vi "01_Main.vi"() -> ()   [LabVIEW 2023]
doc: "This VI shows how to setup and execute a measurement without any user input."
panel:
  out "Loop Counter":i32
  out "size(s)":i32[](array[numeric])
  in  "Fahrprofil Datei":path
  out "IP-Adresse Antrieb":string="192.168.10.5"
  in  "BETRIEBSART ANTRIEB":bool
  in  "Motoren":bool
  out "Digital Antrieb":dbl
  out "Drehmoment Antrieb":dbl
  out "Status/Fehler Antrieb":dbl
  out "Istgeschwindigkeit Antrieb":dbl
  in  "Digital Antrieb":dbl
  in  "Deceleration Antrieb":dbl
  in  "Acceleration Antrieb":dbl
  in  "Speed Antrieb":dbl
  out "IP-Adresse Last":string
  out "Digital":dbl
  out "Drehmoment":dbl
  out "Status/Fehler":dbl
  out "Istgeschwindigkeit":dbl
  in  "Digital A":dbl
  in  "Deceleration":dbl
  in  "Acceleration":dbl
  in  "Speed":dbl
  out "Reserviert":bool
  out "SWES inaktiv":bool
  out "Geschwindigkeit erreicht":bool
  out "Warnung":bool
  out "Fehler":bool
  out "in Position":bool
  out "Relativposition übernommen":bool
  out "Motor dreht":bool
  out "Bremse geöffnet":bool
  out "Endstufenfreigabe":bool
  out "STO inaktiv":bool
  out "Betriebsbereit":bool
  out "Reserviert 8":bool
  out "SWES inaktiv 2":bool
  out "Geschwindigkeit erreicht 2":bool
  out "Warnung 2":bool
  out "Fehler 2":bool
  out "in Position 2":bool
  out "Relativposition übernommen 2":bool
  out "Motor dreht 2":bool
  out "Bremse geöffnet 2":bool
  out "Endstufenfreigabe 2":bool
  out "STO inaktiv 2":bool
  out "Betriebsbereit 2":bool
  in  "Reserviert 9":bool
  in  "Reservier 2":bool
  in  "Reserviert 10":bool
  in  "Reserviert 11":bool
  in  "Reserviert 12":bool
  in  "Reserviert 13":bool
  in  "Reserviert 14":bool
  in  "Reserviert 2":bool
  in  "Reservier":bool
  in  "Reserviert 3":bool
  in  "Reserviert 4":bool
  in  "Reserviert 5":bool
  in  "Reserviert 6":bool
  in  "Reserviert 7":bool
  in  "Bedienelemente - Lastmotor":enum32{"Standard", "Versteckt"}(tab)
  in  "Enable/EmergencyStop Antrieb":bool
  in  "Fehler_Reset Antrieb":bool
  in  "Start L":bool
  in  "Enable/ApplicationStop Antrieb":bool
  in  "Inhibit L":bool
  in  "Standby Antrieb":bool
  in  "Handshake Antrieb":bool
  in  "AS2 aktivieren Antrieb":bool
  in  "Bremse öffnen Antrieb":bool
  out "Standby aktiv 2":bool
  out "AS2 aktiv 2":bool
  out "Handshake 3":bool
  out "referenziert 2":bool
  in  "Bedienelemente - Antriebsmotor":enum32{"Standard", "Versteckt"}(tab)
  in  "Enable/EmergencyStop":bool
  in  "Enable/ApplicationStop":bool
  in  "Fehler_Reset":bool
  in  "Start":bool
  in  "Inhibit":bool
  in  "Standby":bool
  in  "Handshake 2":bool
  in  "AS2 aktivieren":bool
  in  "Bremse öffnen":bool
  out "AS2 aktiv":bool
  out "Handshake":bool
  out "Standby aktiv":bool
  out "referenziert":bool
  out "Numeric":i32
  out "VI wird beendet":string
  in  "VI-Stopp":bool
  out "Diagram 2":waveform(dbl)(graph)
  in  "Kanal 2":i32=2 min=1 max=4 step=1
  in  "Kanal":i32=1 min=1 max=4 step=1
  in  "Datei-Pfad":path
  out "Diagram":waveform(dbl)(graph)
  in  "Messung":bool=TRUE
  out "HBM Driver\nLicense is valid":bool
  # "Betriebsart des Antrieb-Motors wählen; Wenn ein Fahrprofil geladen werden soll dieses über die Datei-Auswahl auswählen. \n\nDanach die Ansteuerung der Motoren mit BETRIEBSART BESTÄTIGEN starten."
  # "Handbetrieb"
  # "Fahrprofil laden"
  # "Manuelle Ansteuerung des Last-Motors"
  # "Manuelle Ansteuerung des Antrieb-Motors"
  # "Datenaquise mit dem HBM Messverstärker"
  # "Messung mit START starten.\n\nWenn die Messdaten gespeichert werden sollen, muss vor \ndem Starten der Messung ein gültiger Dateipfad angegeben werden."
  # "Datenaufzeichnung"
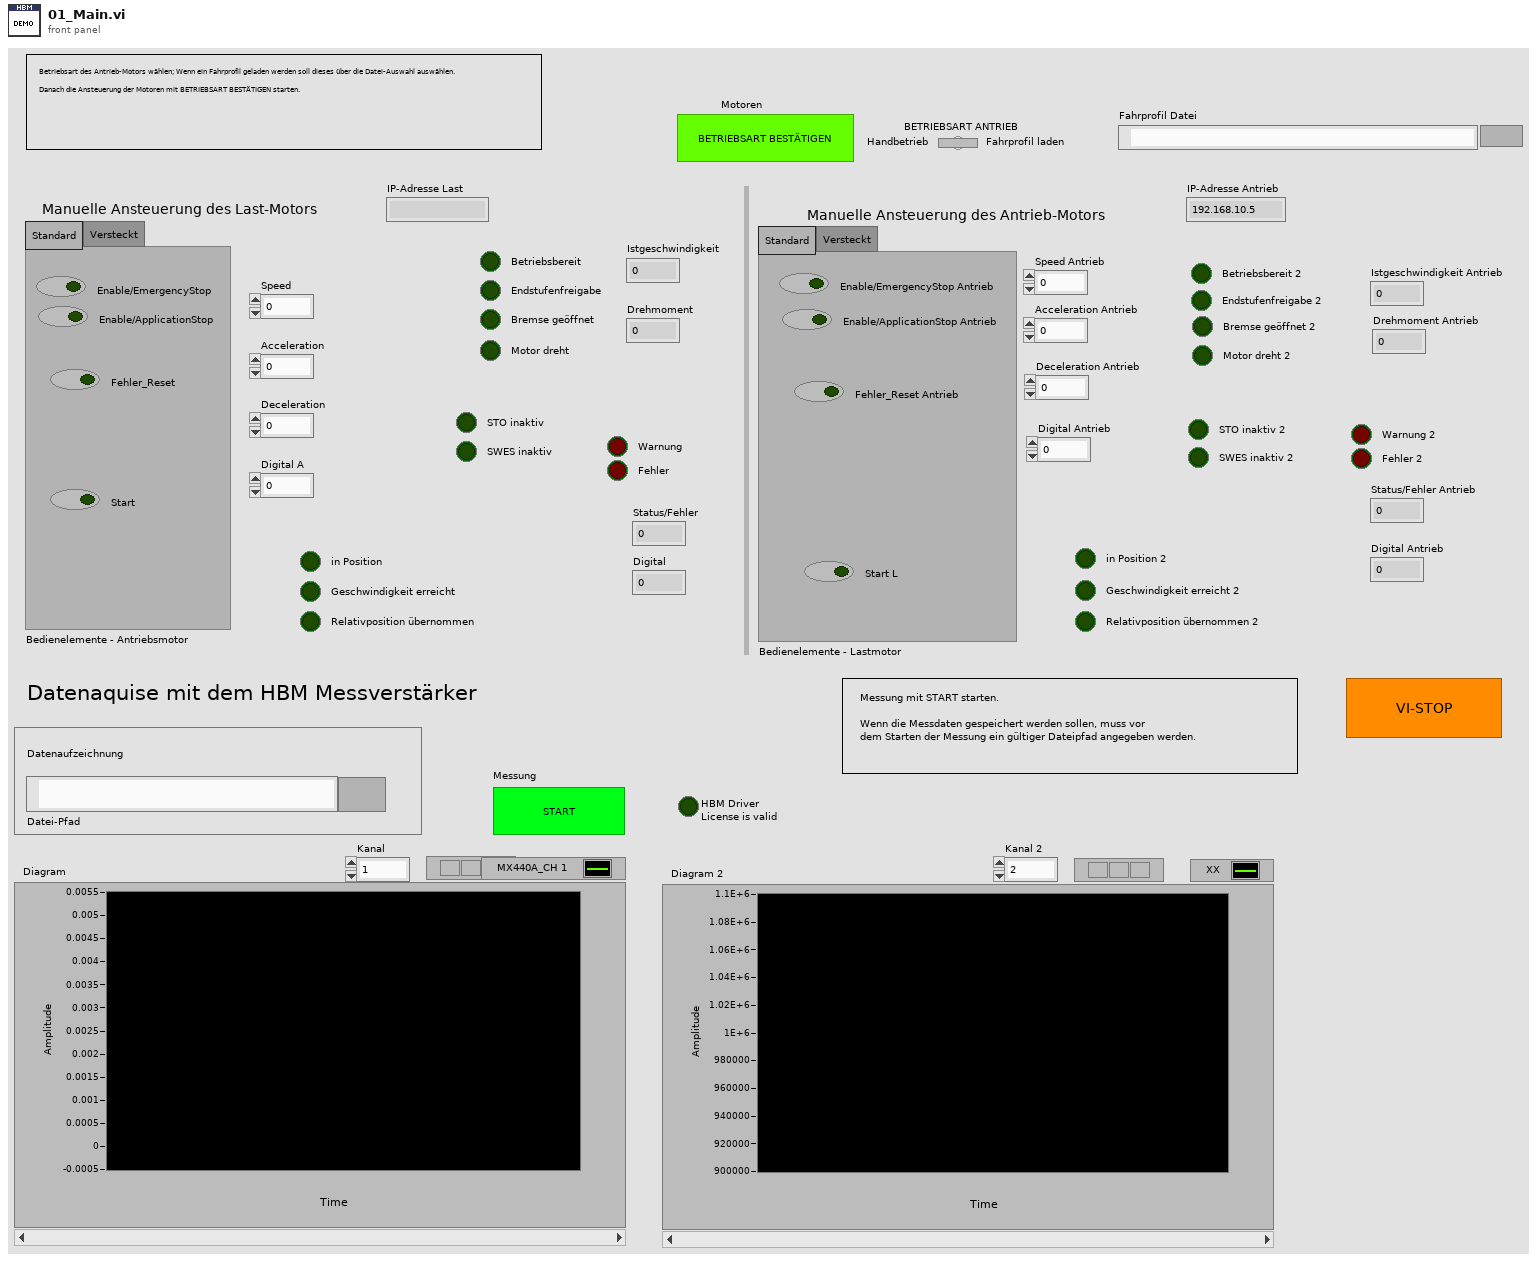
[diagram p1: front panel]
types:
  T1 = cluster{"Devices":refnum<k24>[], "Signals":refnum<k24>[]}
  T2 = enum16{"open", "replace", "create", "open or create", "replace or create", "replace or create with confirmation"}
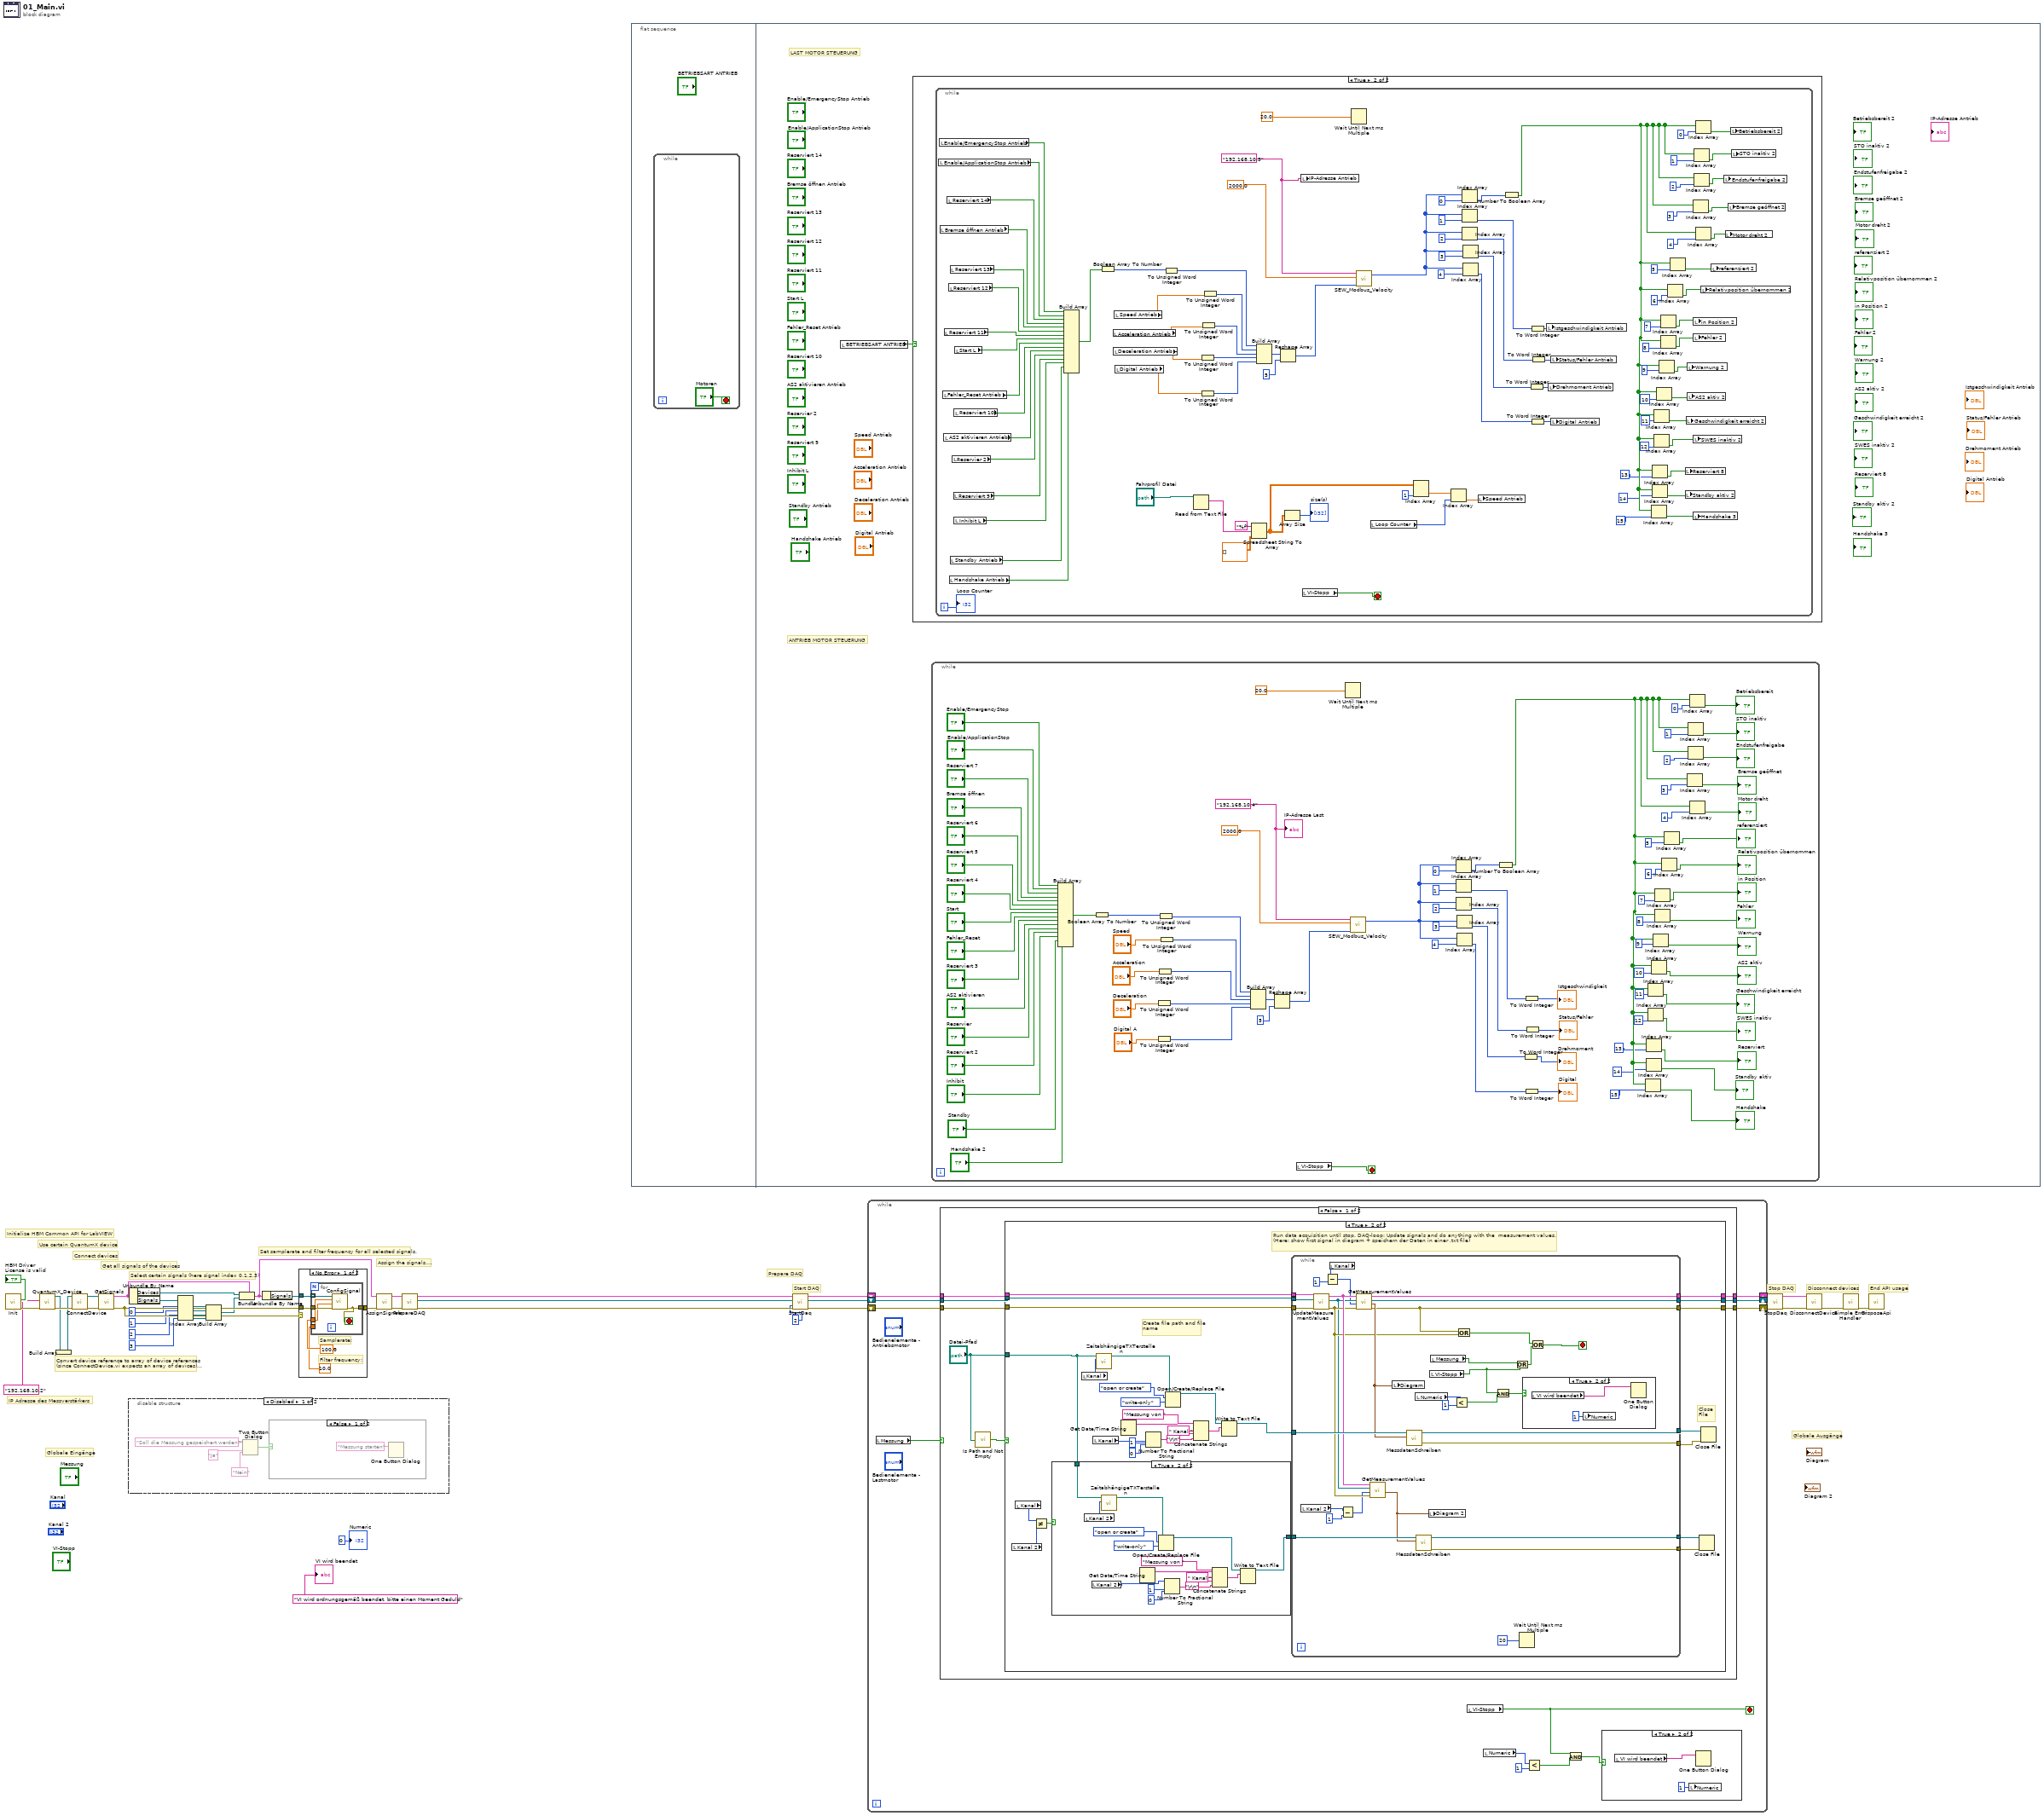
[diagram p0: block diagram]
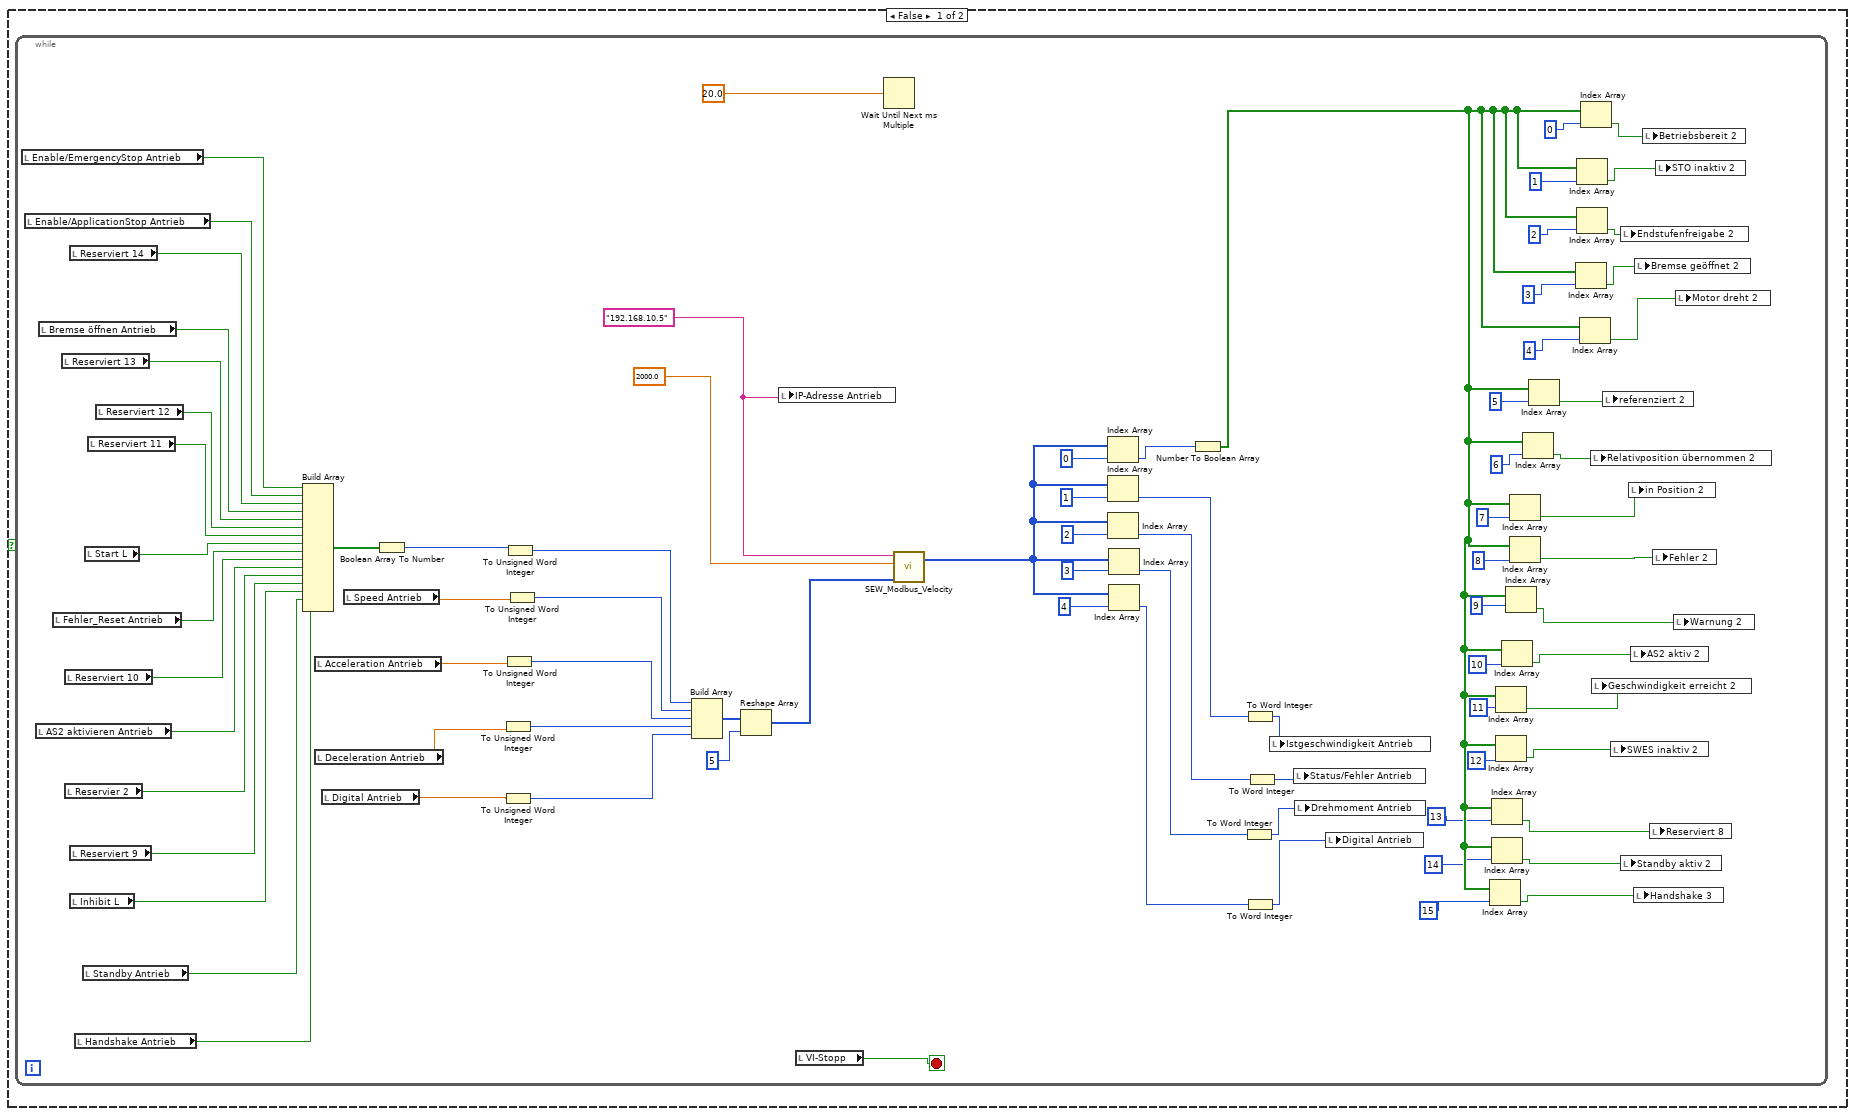
[diagram p2: hidden frame]
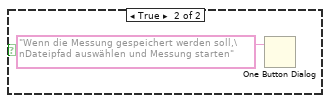
[diagram p3: hidden frame]
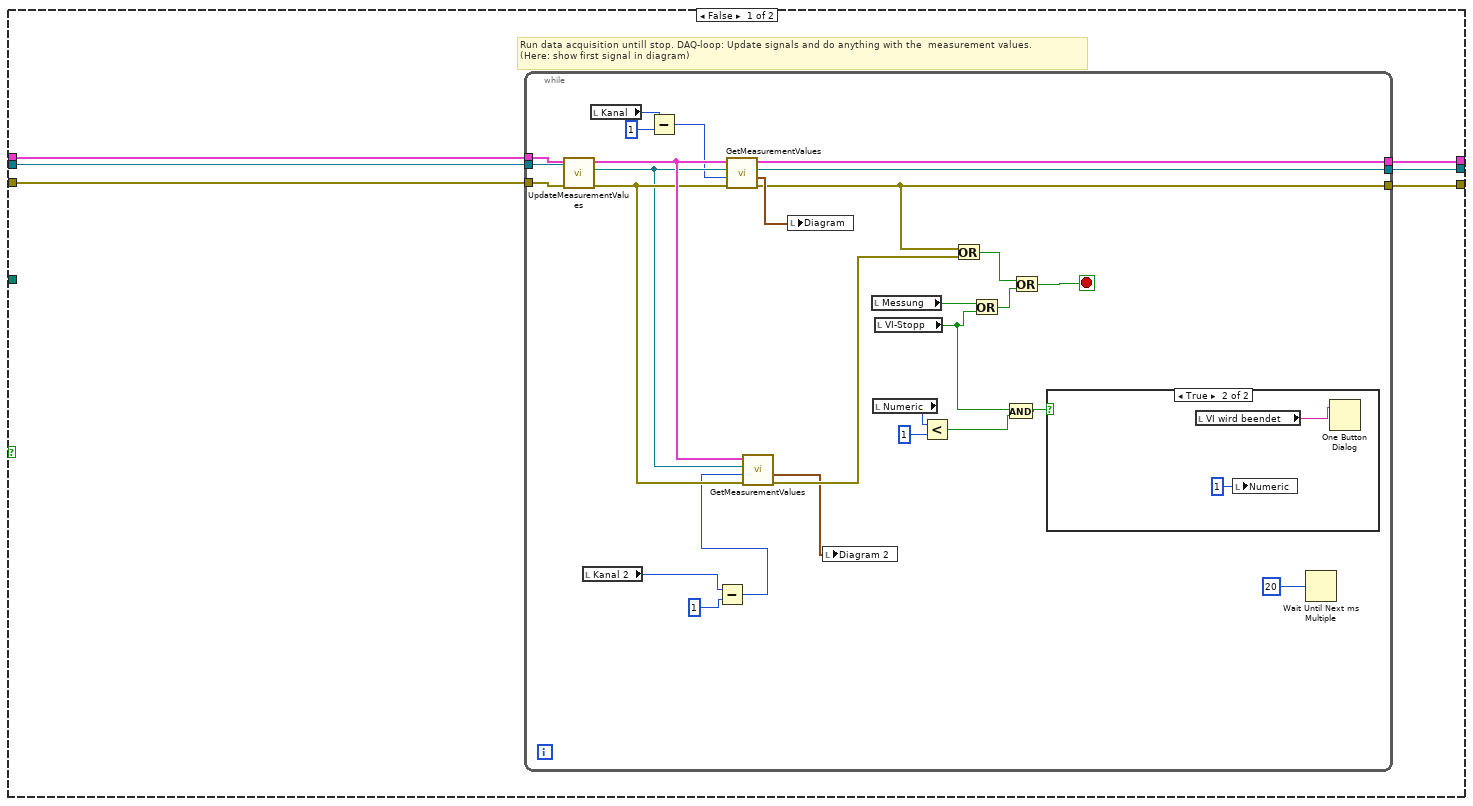
[diagram p6: hidden frame]
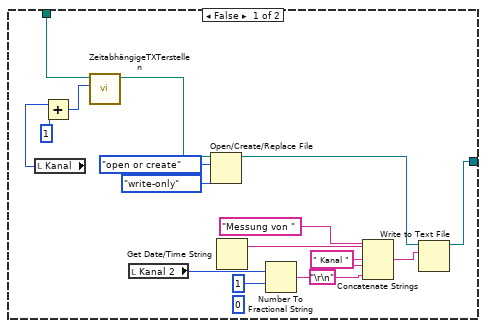
[diagram p8: hidden frame]
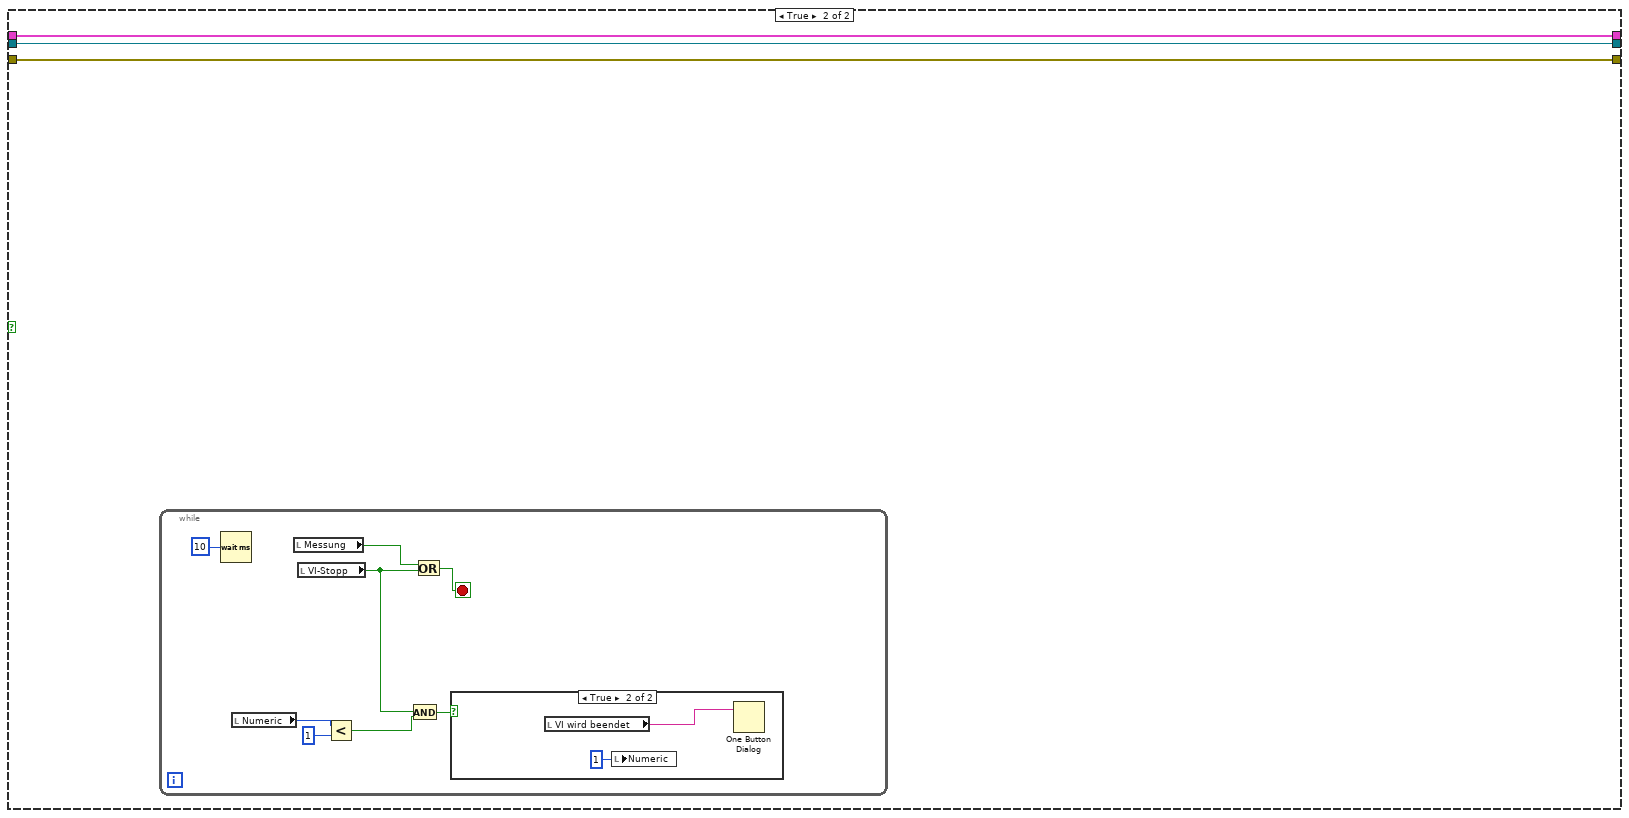
[diagram p10: hidden frame]
diagram:
  # "Globale Ausgänge"
  # "Globale Eingänge"
  # "IP Adresse des Messverstärkers"
  # "Convert device reference to array of device references\n(since ConnectDevice.vi expects an array of devices)..."
  # "Disconnect devices"
  # "Set samplerate and filter frequency for all selected signals."
  # "Initialize HBM Common API for LabVIEW"
  # "End API usage"
  # "Stop DAQ"
  # "Start DAQ"
  # "Prepare DAQ"
  # "Select certain signals (here signal index 0,1,2,3)"
  # "Get all signals of the devices"
  # "Connect devices"
  # "Use certain QuantumX device"
  # "Assign the signals...."
  n1 = call "Init.vi"() -> ("LicenseIsValid"=→"HBM Driver\nLicense is valid":bool, "Error out"=w12:errorcluster)  [unwired: 8 in, 1 out]
  n2 = call "QuantumX_Device.vi"("Error in"=w12, "IPAddress"="192.168.10.2" ("IPAddress of QuantumX device")) -> ("Error out"=w13:errorcluster, "Device"=w10:refnum<k24>)  [unwired: 6 in]
  n3 = Build Array(w10) -> (w9:refnum<k24>[])
  n4 = call "ConnectDevice.vi"("Error in"=w13, "Devices"=w9) -> ("Error out"=w35:errorcluster, "Devices"=w34:refnum<k24>[])  [unwired: 7 in, 1 out]
  n5 = call "GetSignals.vi"("Error in"=w35, "Devices"=w34) -> ("Error out"=w29:errorcluster, "DevicesAndSignals"=w30:T1)  [unwired: 8 in]
  n6 = disable-structure shown="Disabled" {
    frame Disabled {
      n7 = Two Button Dialog(message="Soll die Messung gespeichert werden?", 1:"Nein" ("F button name (\"Cancel\")"), 2:"Ja" ("T button name (\"OK\")")) -> (T button?=w46:bool)
      n8 = case shown="False" w46 {
        frame False {
          n9 = One Button Dialog(message="Messung starten") -> ()  [unwired: 1 in, 1 out]
        }
        frame True {
          n10 = One Button Dialog(message="Wenn die Messung gespeichert werden soll,\nDateipfad auswählen und Messung starten") -> ()  [unwired: 1 in, 1 out]
        }
      }
    }
    frame Enabled {
    }
  }
  n11 = Unbundle By Name(w30) -> ("Devices"=w23:refnum<k24>[], "Signals"=w27:refnum<k24>[])
  n12 = Index Array(array=w27, index #1=0 ("Index"), index #2=1 ("Index"), index #3=2 ("Index"), index #4=3 ("Index")) -> (element #1=w26:refnum<k24>, element #2=w25:refnum<k24>, element #3=w18:refnum<k24>, element #4=w17:refnum<k24>)
  n13 = Build Array(w26, w25, w18, w17) -> (w24:refnum<k24>[])
  n14 = Bundle(cluster=w30, "Devices"=w23, "Signals"=w24) -> (w31:T1)
  n15 = Unbundle By Name(w31) -> ("Signals"=w42:refnum<k24>[])
  n16 = case shown="No Error" w29 {
    tunnel: w29 -> [w53 w59]
    tunnel: w42 -> [w52 _]
    tunnel: [w51 w59] -> w41
    frame No Error {
      # "Filter frequency:"
      # "Samplerate:"
      n17 = for {
        tunnel: w53 -> [w58]
        tunnel: 100.0 ("SampleRate") -> [w57]
        tunnel: 10.0 ("FilterFrequency") -> [w56]
        tunnel: w52 -> [w55] mode=indexing
        tunnel: [w54] -> w51
        stop <- w54 stop-if-true
        n18 = call "ConfigSignal.vi"("Error in"=w58, "SampleRate"=w57, "FilterFrequency"=w56, "Signal"=w55) -> ("Error out"=w54:errorcluster)  [unwired: 7 in]
      }
    }
    frame Error {
    }
  }
  n19 = call "AssignSignals.vi"("Error in"=w41, "DevicesAndSignals"=w31) -> ("Error out"=w39:errorcluster, "DevicesAndSignals"=w40:T1)  [unwired: 8 in]
  n20 = call "PrepareDAQ.vi"("Error in"=w39, "DevicesAndSignals"=w40) -> ("Error out"=w36:errorcluster, "DaqMeasurement"=w37:refnum<k24>, "DevicesAndSignals"=w38:T1)  [unwired: 7 in]
  n21 = flat-sequence {
    frame #0 {
      n22 = while {
        stop <- "Motoren" stop-if-true
      }
    }
    frame #1 {
      # "ANTRIEB MOTOR STEUERUNG"
      # "LAST MOTOR STEUERUNG"
      n23 = local read "BETRIEBSART ANTRIEB"() -> (w61:bool)
      n24 = case shown="True" w61 {
        frame False {
          n25 = while {
            stop <- w103 stop-if-true
            w62 = "192.168.10.5"
            n26 = local read "Enable/EmergencyStop Antrieb"() -> (w86:bool)
            n27 = local read "Enable/ApplicationStop Antrieb"() -> (w85:bool)
            n28 = local read "AS2 aktivieren Antrieb"() -> (w75:bool)
            n29 = local read "Bremse öffnen Antrieb"() -> (w83:bool)
            n30 = local read "Fehler_Reset Antrieb"() -> (w74:bool)
            n31 = local read "Reserviert 13"() -> (w82:bool)
            n32 = local read "Reserviert 10"() -> (w77:bool)
            n33 = local read "Reservier 2"() -> (w76:bool)
            n34 = local read "Reserviert 14"() -> (w84:bool)
            n35 = local read "Reserviert 9"() -> (w78:bool)
            n36 = local read "Inhibit L"() -> (w79:bool)
            n37 = local read "Handshake Antrieb"() -> (w81:bool)
            n38 = local read "Standby Antrieb"() -> (w80:bool)
            n39 = local read "Start L"() -> (w73:bool)
            n40 = local read "Reserviert 11"() -> (w72:bool)
            n41 = local read "Reserviert 12"() -> (w71:bool)
            n42 = Build Array(w86, w85, w84, w83, w82, w71, w72, w73, w74, w77, w75, w76, w78, w79, w80, w81) -> (w136:bool[])
            n43 = local read "Acceleration Antrieb"() -> (w65:dbl)
            n44 = local read "Deceleration Antrieb"() -> (w64:dbl)
            n45 = local read "Digital Antrieb"() -> (w63:dbl)
            n46 = local read "Speed Antrieb"() -> (w66:dbl)
            n47 = Boolean Array To Number(Boolean array=w136) -> (number=w137:u32)
            n48 = To Unsigned Word Integer(number=w64) -> (unsigned 16bit integer=w140:u16)
            n49 = To Unsigned Word Integer(number=w63) -> (unsigned 16bit integer=w141:u16)
            n50 = To Unsigned Word Integer(number=w65) -> (unsigned 16bit integer=w139:u16)
            n51 = To Unsigned Word Integer(number=w137) -> (unsigned 16bit integer=w138:u16)
            n52 = To Unsigned Word Integer(number=w66) -> (unsigned 16bit integer=w142:u16)
            n53 = Build Array(w138, w142, w139, w140, w141) -> (w143:u16[])
            n54 = Reshape Array(w143, 5) -> (w133:u16[])
            n55 = local write "IP-Adresse Antrieb"(w62) -> ()
            n56 = local read "VI-Stopp"() -> (w103:bool)
            n57 = Wait Until Next ms Multiple(millisecond multiple=20.0 ("Update(ms)")) -> ()  [unwired: 1 out]
            n58 = call "SEW_Modbus_Velocity.vi"("Remote IP Address"=w62, "Timeout [ms]"=2000.0 ("Timeout (ms)"), "Output (Write Multiple Register) 2"=w133) -> ("Input (Read Holding Register) 2"=w131:u16[])  [unwired: 3 in]
            n59 = Index Array(array=w131, index=0) -> (element=w121:u16)
            n60 = Index Array(array=w131, index=1) -> (element=w122:u16)
            n61 = Index Array(array=w131, index=2) -> (element=w123:u16)
            n62 = Index Array(array=w131, index=3) -> (element=w124:u16)
            n63 = Index Array(array=w131, index=4) -> (element=w125:u16)
            n64 = Number To Boolean Array(number=w121) -> (Boolean array=w120:bool[])
            n65 = To Word Integer(number=w124) -> (16bit integer=w68:i16)
            n66 = To Word Integer(number=w122) -> (16bit integer=w70:i16)
            n67 = To Word Integer(number=w125) -> (16bit integer=w67:i16)
            n68 = To Word Integer(number=w123) -> (16bit integer=w69:i16)
            n69 = local write "Istgeschwindigkeit Antrieb"(w70) -> ()
            n70 = local write "Status/Fehler Antrieb"(w69) -> ()
            n71 = local write "Drehmoment Antrieb"(w68) -> ()
            n72 = local write "Digital Antrieb"(w67) -> ()
            n73 = Index Array(array=w120, index=15) -> (element=w87:bool)
            n74 = Index Array(array=w120, index=13) -> (element=w89:bool)
            n75 = Index Array(array=w120, index=14) -> (element=w88:bool)
            n76 = Index Array(array=w120, index=11) -> (element=w91:bool)
            n77 = Index Array(array=w120, index=12) -> (element=w90:bool)
            n78 = Index Array(array=w120, index=10) -> (element=w92:bool)
            n79 = Index Array(array=w120, index=9) -> (element=w93:bool)
            n80 = Index Array(array=w120, index=7) -> (element=w95:bool)
            n81 = Index Array(array=w120, index=8) -> (element=w94:bool)
            n82 = Index Array(array=w120, index=6) -> (element=w96:bool)
            n83 = Index Array(array=w120, index=5) -> (element=w97:bool)
            n84 = Index Array(array=w120, index=3) -> (element=w99:bool)
            n85 = Index Array(array=w120, index=1) -> (element=w101:bool)
            n86 = Index Array(array=w120, index=2) -> (element=w100:bool)
            n87 = Index Array(array=w120, index=4) -> (element=w98:bool)
            n88 = Index Array(array=w120, index=0) -> (element=w102:bool)
            n89 = local write "Relativposition übernommen 2"(w96) -> ()
            n90 = local write "Geschwindigkeit erreicht 2"(w91) -> ()
            n91 = local write "referenziert 2"(w97) -> ()
            n92 = local write "SWES inaktiv 2"(w90) -> ()
            n93 = local write "Endstufenfreigabe 2"(w100) -> ()
            n94 = local write "Standby aktiv 2"(w88) -> ()
            n95 = local write "in Position 2"(w95) -> ()
            n96 = local write "AS2 aktiv 2"(w92) -> ()
            n97 = local write "Handshake 3"(w87) -> ()
            n98 = local write "Bremse geöffnet 2"(w99) -> ()
            n99 = local write "Betriebsbereit 2"(w102) -> ()
            n100 = local write "Reserviert 8"(w89) -> ()
            n101 = local write "Fehler 2"(w94) -> ()
            n102 = local write "STO inaktiv 2"(w101) -> ()
            n103 = local write "Warnung 2"(w93) -> ()
            n104 = local write "Motor dreht 2"(w98) -> ()
          }
        }
        frame True {
          n105 = while {
            i -> [w146]
            stop <- w196 stop-if-true
            w155 = "192.168.10.5"
            n106 = local read "Enable/ApplicationStop Antrieb"() -> (w177:bool)
            n107 = local read "Enable/EmergencyStop Antrieb"() -> (w176:bool)
            n108 = local read "Bremse öffnen Antrieb"() -> (w179:bool)
            n109 = local read "Fehler_Reset Antrieb"() -> (w184:bool)
            n110 = local read "AS2 aktivieren Antrieb"() -> (w186:bool)
            n111 = local read "Reserviert 11"() -> (w182:bool)
            n112 = local read "Reserviert 14"() -> (w178:bool)
            n113 = local read "Reserviert 12"() -> (w181:bool)
            n114 = local read "Handshake Antrieb"() -> (w191:bool)
            n115 = local read "Reserviert 13"() -> (w180:bool)
            n116 = local read "Standby Antrieb"() -> (w190:bool)
            n117 = local read "Reservier 2"() -> (w187:bool)
            n118 = local read "Reserviert 9"() -> (w188:bool)
            n119 = local read "Reserviert 10"() -> (w185:bool)
            n120 = local read "Inhibit L"() -> (w189:bool)
            n121 = local read "Start L"() -> (w183:bool)
            n122 = Build Array(w176, w177, w178, w179, w180, w181, w182, w183, w184, w185, w186, w187, w188, w189, w190, w191) -> (w229:bool[])
            n123 = Boolean Array To Number(Boolean array=w229) -> (number=w230:u32)
            n124 = local read "Acceleration Antrieb"() -> (w194:dbl)
            n125 = local read "Deceleration Antrieb"() -> (w193:dbl)
            n126 = local read "Speed Antrieb"() -> (w195:dbl)
            n127 = local read "Digital Antrieb"() -> (w192:dbl)
            n128 = To Unsigned Word Integer(number=w230) -> (unsigned 16bit integer=w231:u16)
            n129 = Read from Text File(file (use dialog)="Fahrprofil Datei") -> (text=w152:string)  [unwired: 2 in, 4 out]
            n130 = To Unsigned Word Integer(number=w193) -> (unsigned 16bit integer=w233:u16)
            n131 = To Unsigned Word Integer(number=w192) -> (unsigned 16bit integer=w234:u16)
            n132 = To Unsigned Word Integer(number=w194) -> (unsigned 16bit integer=w232:u16)
            n133 = To Unsigned Word Integer(number=w195) -> (unsigned 16bit integer=w235:u16)
            n134 = Spreadsheet String To Array(format string="%f", spreadsheet string=w152, array type (2D Dbl)=dbl[][] []) -> (array=w147:dbl[][])  [unwired: 1 in]
            n135 = Build Array(w231, w235, w232, w233, w234) -> (w236:u16[])
            n136 = Reshape Array(w236, 5) -> (w226:u16[])
            n137 = Array Size(array=w147) -> (size(s)=→"size(s)":i32[])
            n138 = local write "IP-Adresse Antrieb"(w155) -> ()
            n139 = local read "VI-Stopp"() -> (w196:bool)
            n140 = Wait Until Next ms Multiple(millisecond multiple=20.0 ("Update(ms)")) -> ()  [unwired: 1 out]
            n141 = call "SEW_Modbus_Velocity.vi"("Remote IP Address"=w155, "Timeout [ms]"=2000.0 ("Timeout (ms)"), "Output (Write Multiple Register) 2"=w226) -> ("Input (Read Holding Register) 2"=w224:u16[])  [unwired: 3 in]
            n142 = local read "Loop Counter"() -> (w145:i32)
            n143 = Index Array(array=w147, index (col)=1 ("disabled index (col)")) -> (element=w154:dbl[])  [unwired: 1 in]
            n144 = Index Array(array=w154, index=w145) -> (element=w144:dbl)
            n145 = Index Array(array=w224, index=0) -> (element=w214:u16)
            n146 = Index Array(array=w224, index=1) -> (element=w215:u16)
            n147 = Index Array(array=w224, index=2) -> (element=w216:u16)
            n148 = Index Array(array=w224, index=3) -> (element=w217:u16)
            n149 = Index Array(array=w224, index=4) -> (element=w218:u16)
            n150 = local write "Speed Antrieb"(w144) -> ()
            n151 = Number To Boolean Array(number=w214) -> (Boolean array=w213:bool[])
            n152 = To Word Integer(number=w217) -> (16bit integer=w173:i16)
            n153 = To Word Integer(number=w215) -> (16bit integer=w175:i16)
            n154 = To Word Integer(number=w218) -> (16bit integer=w172:i16)
            n155 = To Word Integer(number=w216) -> (16bit integer=w174:i16)
            n156 = local write "Istgeschwindigkeit Antrieb"(w175) -> ()
            n157 = local write "Drehmoment Antrieb"(w173) -> ()
            n158 = local write "Status/Fehler Antrieb"(w174) -> ()
            n159 = local write "Digital Antrieb"(w172) -> ()
            n160 = Index Array(array=w213, index=15) -> (element=w171:bool)
            n161 = Index Array(array=w213, index=13) -> (element=w169:bool)
            n162 = Index Array(array=w213, index=14) -> (element=w170:bool)
            n163 = Index Array(array=w213, index=11) -> (element=w167:bool)
            n164 = Index Array(array=w213, index=12) -> (element=w168:bool)
            n165 = Index Array(array=w213, index=10) -> (element=w166:bool)
            n166 = Index Array(array=w213, index=9) -> (element=w165:bool)
            n167 = Index Array(array=w213, index=7) -> (element=w163:bool)
            n168 = Index Array(array=w213, index=8) -> (element=w164:bool)
            n169 = Index Array(array=w213, index=6) -> (element=w162:bool)
            n170 = Index Array(array=w213, index=5) -> (element=w161:bool)
            n171 = local write "Reserviert 8"(w169) -> ()
            n172 = local write "Standby aktiv 2"(w170) -> ()
            n173 = local write "Geschwindigkeit erreicht 2"(w167) -> ()
            n174 = local write "Warnung 2"(w165) -> ()
            n175 = local write "AS2 aktiv 2"(w166) -> ()
            n176 = local write "SWES inaktiv 2"(w168) -> ()
            n177 = local write "Handshake 3"(w171) -> ()
            n178 = Index Array(array=w213, index=3) -> (element=w159:bool)
            n179 = local write "in Position 2"(w163) -> ()
            n180 = local write "Fehler 2"(w164) -> ()
            n181 = Index Array(array=w213, index=1) -> (element=w157:bool)
            n182 = Index Array(array=w213, index=2) -> (element=w158:bool)
            n183 = Index Array(array=w213, index=4) -> (element=w160:bool)
            n184 = Index Array(array=w213, index=0) -> (element=w156:bool)
            n185 = local write "Relativposition übernommen 2"(w162) -> ()
            n186 = local write "referenziert 2"(w161) -> ()
            n187 = local write "Endstufenfreigabe 2"(w158) -> ()
            n188 = local write "Motor dreht 2"(w160) -> ()
            n189 = local write "Bremse geöffnet 2"(w159) -> ()
            n190 = local write "Betriebsbereit 2"(w156) -> ()
            n191 = local write "STO inaktiv 2"(w157) -> ()
            "Loop Counter" <- w146
          }
        }
      }
      n192 = while {
        stop <- w278 stop-if-true
        w277 = "192.168.10.4"
        n193 = Build Array("Enable/EmergencyStop", "Enable/ApplicationStop", "Reserviert 7", "Bremse öffnen", "Reserviert 6", "Reserviert 5", "Reserviert 4", "Start", "Fehler_Reset", "Reserviert 3", "AS2 aktivieren", "Reservier", "Reserviert 2", "Inhibit", "Standby", "Handshake 2") -> (w311:bool[])
        n194 = Boolean Array To Number(Boolean array=w311) -> (number=w312:u32)
        n195 = To Unsigned Word Integer(number="Deceleration") -> (unsigned 16bit integer=w315:u16)
        n196 = To Unsigned Word Integer(number="Digital A") -> (unsigned 16bit integer=w316:u16)
        n197 = To Unsigned Word Integer(number="Acceleration") -> (unsigned 16bit integer=w314:u16)
        n198 = To Unsigned Word Integer(number=w312) -> (unsigned 16bit integer=w313:u16)
        n199 = To Unsigned Word Integer(number="Speed") -> (unsigned 16bit integer=w317:u16)
        n200 = Build Array(w313, w317, w314, w315, w316) -> (w318:u16[])
        n201 = Reshape Array(w318, 5) -> (w308:u16[])
        n202 = local read "VI-Stopp"() -> (w278:bool)
        n203 = Wait Until Next ms Multiple(millisecond multiple=20.0 ("Update(ms)")) -> ()  [unwired: 1 out]
        n204 = call "SEW_Modbus_Velocity.vi"("Remote IP Address"=w277, "Timeout [ms]"=2000.0 ("Timeout (ms)"), "Output (Write Multiple Register) 2"=w308) -> ("Input (Read Holding Register) 2"=w306:u16[])  [unwired: 3 in]
        n205 = Index Array(array=w306, index=0) -> (element=w296:u16)
        n206 = Index Array(array=w306, index=1) -> (element=w297:u16)
        n207 = Index Array(array=w306, index=2) -> (element=w298:u16)
        n208 = Index Array(array=w306, index=3) -> (element=w299:u16)
        n209 = Index Array(array=w306, index=4) -> (element=w300:u16)
        n210 = Number To Boolean Array(number=w296) -> (Boolean array=w295:bool[])
        n211 = To Word Integer(number=w299) -> (16bit integer=→"Drehmoment":i16)
        n212 = To Word Integer(number=w297) -> (16bit integer=→"Istgeschwindigkeit":i16)
        n213 = To Word Integer(number=w300) -> (16bit integer=→"Digital":i16)
        n214 = To Word Integer(number=w298) -> (16bit integer=→"Status/Fehler":i16)
        n215 = Index Array(array=w295, index=15) -> (element=→"Handshake":bool)
        n216 = Index Array(array=w295, index=13) -> (element=→"Reserviert":bool)
        n217 = Index Array(array=w295, index=14) -> (element=→"Standby aktiv":bool)
        n218 = Index Array(array=w295, index=11) -> (element=→"Geschwindigkeit erreicht":bool)
        n219 = Index Array(array=w295, index=12) -> (element=→"SWES inaktiv":bool)
        n220 = Index Array(array=w295, index=10) -> (element=→"AS2 aktiv":bool)
        n221 = Index Array(array=w295, index=9) -> (element=→"Warnung":bool)
        n222 = Index Array(array=w295, index=7) -> (element=→"in Position":bool)
        n223 = Index Array(array=w295, index=8) -> (element=→"Fehler":bool)
        n224 = Index Array(array=w295, index=6) -> (element=→"Relativposition übernommen":bool)
        n225 = Index Array(array=w295, index=5) -> (element=→"referenziert":bool)
        n226 = Index Array(array=w295, index=3) -> (element=→"Bremse geöffnet":bool)
        n227 = Index Array(array=w295, index=1) -> (element=→"STO inaktiv":bool)
        n228 = Index Array(array=w295, index=2) -> (element=→"Endstufenfreigabe":bool)
        n229 = Index Array(array=w295, index=4) -> (element=→"Motor dreht":bool)
        n230 = Index Array(array=w295, index=0) -> (element=→"Betriebsbereit":bool)
        "IP-Adresse Last" <- w277
      }
    }
  }
  n231 = call "StartDaq.vi"("DevicesAndSignals"=w38, "DaqMeasurement"=w37, "AcquisitionMode"=2, "Error in"=w36) -> ("DevicesAndSignals"=w5:T1, "DaqMeasurement"=w4:refnum<k24>, "Error out"=w3:errorcluster)  [unwired: 7 in, 2 out]
  n232 = while {
    shift-right: [w330] -> w7
    shift-left: w5 -> [w328]
    shift-right: [w324] -> w8
    shift-left: w4 -> [w327]
    shift-right: [w329] -> w6
    shift-left: w3 -> [w326]
    stop <- w320 stop-if-true
    n233 = local read "Messung"() -> (w325:bool)
    n234 = case shown="False" w325 {
      tunnel: [w339 w477] -> w330
      tunnel: [w338 w475] -> w329
      tunnel: w328 -> [w337 w477]
      tunnel: w327 -> [w336 w476]
      tunnel: w326 -> [w335 w475]
      tunnel: [w340 w476] -> w324
      frame False {
        n235 = call <vilib>:"Is Path and Not Empty.vi"("path"="Datei-Pfad") -> ("Is Path and Not Empty?"=w333:bool)  [unwired: 4 in]
        n236 = case shown="True" w333 {
          tunnel: [w342 w404] -> w340
          tunnel: [w343 w403] -> w339
          tunnel: [w341 w402] -> w338
          tunnel: w337 -> [w346 w401]
          tunnel: w336 -> [w345 w400]
          tunnel: w335 -> [w344 w399]
          tunnel: "Datei-Pfad" -> [_ w395]
          frame False {
            # "Run data acquisition untill stop. DAQ-loop: Update signals and do anything with the  measurement values.\n(Here: show first signal in diagram)"
            n237 = while {
              tunnel: [w374] -> w342
              tunnel: [w373] -> w343
              tunnel: [w366] -> w341
              tunnel: w346 -> [w371]
              tunnel: w345 -> [w370]
              tunnel: w344 -> [w369]
              stop <- w352 stop-if-true
              n238 = call "UpdateMeasurementValues.vi"("Error in"=w369, "DaqMeasurement"=w370, "DevicesAndSignals"=w371) -> ("Error out"=w364:errorcluster, "DaqMeasurement"=w363:refnum<k24>, "DevicesAndSignals"=w365:T1)  [unwired: 6 in]
              n239 = local read "Kanal 2"() -> (w356:i32)
              n240 = local read "Kanal"() -> (w359:i32)
              n241 = Subtract(x=w359, y=1) -> (x-y=w358:i32)
              n242 = Subtract(x=w356, y=1) -> (x-y=w355:i32)
              n243 = call "GetMeasurementValues.vi"("Error in"=w364, "Index"=w358, "DaqMeasurement"=w363, "DevicesAndSignals"=w365) -> ("Error out"=w366:errorcluster, "Waveform"=w368:waveform(dbl), "DaqMeasurement"=w374:refnum<k24>, "DevicesAndSignals"=w373:T1)  [unwired: 2 in, 2 out]
              n244 = call "GetMeasurementValues.vi"("Error in"=w364, "Index"=w355, "DaqMeasurement"=w363, "DevicesAndSignals"=w365) -> ("Error out"=w362:errorcluster, "Waveform"=w361:waveform(dbl))  [unwired: 2 in, 4 out]
              n245 = local write "Diagram"(w368) -> ()
              n246 = local write "Diagram 2"(w361) -> ()
              n247 = local read "Messung"() -> (w353:bool)
              n248 = local read "Numeric"() -> (w347:i32)
              n249 = local read "VI-Stopp"() -> (w349:bool)
              n250 = Less?(x=w347, y=1) -> (x < y?=w350:bool)
              n251 = Or(x=w366, y=w362) -> (x .or. y?=w367:bool)
              n252 = Or(x=w353, y=w349) -> (x .or. y?=w354:bool)
              n253 = And(x=w349, y=w350) -> (x .and. y?=w348:bool)
              n254 = Or(x=w367, y=w354) -> (x .or. y?=w352:bool)
              n255 = case shown="True" w348 {
                frame False {
                }
                frame True {
                  n256 = local read "VI wird beendet"() -> (w376:string)
                  n257 = local write "Numeric"(1 ("Numeric")) -> ()
                  n258 = One Button Dialog(message=w376) -> ()  [unwired: 1 in, 1 out]
                }
              }
              n259 = Wait Until Next ms Multiple(millisecond multiple=u32 20 ("Vielfache von ms")) -> ()  [unwired: 1 out]
            }
          }
          frame True {
            # "Close\nFile"
            # "Create file path and file name"
            # "Run data acquisition until stop. DAQ-loop: Update signals and do anything with the  measurement values.\n(Here: show first signal in diagram + speichern der Daten in einer .txt file)"
            n260 = local read "Kanal 2"() -> (w388:i32)
            n261 = local read "Kanal"() -> (w389:i32)
            n262 = Not Equal?(x=w389, y=w388) -> (x != y?=w390:bool)
            n263 = case shown="True" w390 {
              tunnel: w395 -> [w423 w437]
              tunnel: [w407 w425] -> w392
              frame False {
                (unwired) i16 0 ("precision (6)")
                n264 = local read "Kanal"() -> (w421:i32)
                n265 = Add(x=w421, y=1) -> (x+y=w422:i32)
                n266 = call "ZeitabhängigeTXTerstellen.vi"("Signal index to display"=w422, "path"=w423) -> ("Path"=w419:path)  [unwired: 9 in]
                n267 = local read "Kanal 2"() -> (w408:i32)
                n268 = Open/Create/Replace File(file path (use dialog)=w419, operation (0:open)=T2."open or create", access (0:read/write)=enum16{"read/write", "read-only", "write-only"}."write-only") -> (refnum out=w409:refnum<file>)  [unwired: 3 in, 2 out]
                n269 = Get Date/Time String() -> (date string=w415:string)  [unwired: 3 in, 1 out]
                n270 = Number To Fractional String(number=w408, width (-)=i16 1) -> (F-format string=w411:string)  [unwired: 2 in]
                n271 = Concatenate Strings("Messung von " ("text"), w415, " Kanal " ("string"), w411, "\r\n") -> (w414:string)
                n272 = Write to Text File(file (use dialog)=w409, text=w414) -> (refnum out=w407:refnum<file>)  [unwired: 2 in, 2 out]
              }
              frame True {
                n273 = local read "Kanal 2"() -> (w439:i32)
                n274 = local read "Kanal 2"() -> (w427:i32)
                n275 = call "ZeitabhängigeTXTerstellen.vi"("Signal index to display"=w439, "path"=w437) -> ("Path"=w438:path)  [unwired: 9 in]
                n276 = Get Date/Time String() -> (date string=w433:string)  [unwired: 3 in, 1 out]
                n277 = Open/Create/Replace File(file path (use dialog)=w438, operation (0:open)=T2."open or create", access (0:read/write)=enum16{"read/write", "read-only", "write-only"}."write-only") -> (refnum out=w426:refnum<file>)  [unwired: 3 in, 2 out]
                n278 = Number To Fractional String(number=w427, width (-)=i16 1, precision (6)=i16 0) -> (F-format string=w429:string)  [unwired: 1 in]
                n279 = Concatenate Strings("Messung von " ("text"), w433, " Kanal " ("string"), w429, "\r\n") -> (w432:string)
                n280 = Write to Text File(file (use dialog)=w426, text=w432) -> (refnum out=w425:refnum<file>)  [unwired: 2 in, 2 out]
              }
            }
            n281 = local read "Kanal"() -> (w396:i32)
            n282 = local read "Kanal"() -> (w379:i32)
            n283 = call "ZeitabhängigeTXTerstellen.vi"("Signal index to display"=w396, "path"=w395) -> ("Path"=w391:path)  [unwired: 9 in]
            n284 = Get Date/Time String() -> (date string=w386:string)  [unwired: 3 in, 1 out]
            n285 = Number To Fractional String(number=w379, width (-)=i16 1, precision (6)=i16 0) -> (F-format string=w380:string)  [unwired: 1 in]
            n286 = Open/Create/Replace File(file path (use dialog)=w391, operation (0:open)=T2."open or create", access (0:read/write)=enum16{"read/write", "read-only", "write-only"}."write-only") -> (refnum out=w377:refnum<file>)  [unwired: 3 in, 2 out]
            n287 = Concatenate Strings("Messung von " ("text"), w386, " Kanal " ("string"), w380, "\r\n") -> (w385:string)
            n288 = Write to Text File(file (use dialog)=w377, text=w385) -> (refnum out=w384:refnum<file>)  [unwired: 2 in, 2 out]
            n289 = while {
              tunnel: w400 -> [w471]
              tunnel: [w470] -> w404
              tunnel: [w469] -> w403
              tunnel: w399 -> [w472]
              tunnel: [w456] -> w402
              tunnel: [w466] -> w406
              tunnel: [w465] -> w405
              tunnel: w384 -> [w464]
              tunnel: w401 -> [w463]
              tunnel: w392 -> [w458]
              tunnel: [w461] -> w398
              tunnel: [w460] -> w397
              stop <- w467 stop-if-true
              n290 = local read "Kanal 2"() -> (w448:i32)
              n291 = call "UpdateMeasurementValues.vi"("Error in"=w472, "DaqMeasurement"=w471, "DevicesAndSignals"=w463) -> ("Error out"=w455:errorcluster, "DaqMeasurement"=w453:refnum<k24>, "DevicesAndSignals"=w459:T1)  [unwired: 6 in]
              n292 = local read "Kanal"() -> (w452:i32)
              n293 = Subtract(x=w452, y=1) -> (x-y=w450:i32)
              n294 = Subtract(x=w448, y=1) -> (x-y=w447:i32)
              n295 = call "GetMeasurementValues.vi"("Error in"=w455, "Index"=w450, "DaqMeasurement"=w453, "DevicesAndSignals"=w459) -> ("Error out"=w456:errorcluster, "Waveform"=w462:waveform(dbl), "DaqMeasurement"=w470:refnum<k24>, "DevicesAndSignals"=w469:T1)  [unwired: 2 in, 2 out]
              n296 = call "GetMeasurementValues.vi"("Error in"=w455, "Index"=w447, "DaqMeasurement"=w453, "DevicesAndSignals"=w459) -> ("Waveform"=w457:waveform(dbl))  [unwired: 2 in, 5 out]
              n297 = local write "Diagram"(w462) -> ()
              n298 = call "MessdatenSchreiben.vi"("Waveform"=w462, "Byte Stream File in"=w464) -> ("error out"=w466:errorcluster, "Byte Stream File out"=w465:refnum<file>)  [unwired: 8 in]
              n299 = local read "Numeric"() -> (w440:i32)
              n300 = call "MessdatenSchreiben.vi"("Waveform"=w457, "Byte Stream File in"=w458) -> ("error out"=w460:errorcluster, "Byte Stream File out"=w461:refnum<file>)  [unwired: 8 in]
              n301 = local write "Diagram 2"(w457) -> ()
              n302 = local read "VI-Stopp"() -> (w442:bool)
              n303 = local read "Messung"() -> (w445:bool)
              n304 = Less?(x=w440, y=1) -> (x < y?=w443:bool)
              n305 = Or(x=w456, y=w455) -> (x .or. y?=w454:bool)
              n306 = And(x=w442, y=w443) -> (x .and. y?=w441:bool)
              n307 = Or(x=w445, y=w442) -> (x .or. y?=w446:bool)
              n308 = Wait Until Next ms Multiple(millisecond multiple=u32 20 ("Vielfache von ms")) -> ()  [unwired: 1 out]
              n309 = case shown="True" w441 {
                frame False {
                }
                frame True {
                  n310 = local read "VI wird beendet"() -> (w474:string)
                  n311 = local write "Numeric"(1 ("Numeric")) -> ()
                  n312 = One Button Dialog(message=w474) -> ()  [unwired: 1 in, 1 out]
                }
              }
              n313 = Or(x=w454, y=w446) -> (x .or. y?=w467:bool)
            }
            n314 = Close File(refnum=w398, error in=w397) -> ()  [unwired: 2 out]
            n315 = Close File(refnum=w405, error in=w406) -> ()  [unwired: 2 out]
          }
        }
      }
      frame True {
        n316 = while {
          stop <- w483 stop-if-true
          n317 = Wait (ms)(milliseconds to wait=u32 10) -> ()  [unwired: 1 out]
          n318 = local read "Numeric"() -> (w480:i32)
          n319 = local read "Messung"() -> (w484:bool)
          n320 = local read "VI-Stopp"() -> (w481:bool)
          n321 = Less?(x=w480, y=1) -> (x < y?=w478:bool)
          n322 = And(x=w481, y=w478) -> (x .and. y?=w482:bool)
          n323 = Or(x=w484, y=w481) -> (x .or. y?=w483:bool)
          n324 = case shown="True" w482 {
            frame False {
            }
            frame True {
              n325 = local read "VI wird beendet"() -> (w487:string)
              n326 = local write "Numeric"(1 ("Numeric")) -> ()
              n327 = One Button Dialog(message=w487) -> ()  [unwired: 1 in, 1 out]
            }
          }
        }
      }
    }
    n328 = local read "VI-Stopp"() -> (w320:bool)
    n329 = local read "Numeric"() -> (w319:i32)
    n330 = Less?(x=w319, y=1) -> (x < y?=w323:bool)
    n331 = And(x=w320, y=w323) -> (x .and. y?=w321:bool)
    n332 = case shown="True" w321 {
      frame False {
      }
      frame True {
        n333 = local read "VI wird beendet"() -> (w332:string)
        n334 = local write "Numeric"(1 ("Numeric")) -> ()
        n335 = One Button Dialog(message=w332) -> ()  [unwired: 1 in, 1 out]
      }
    }
  }
  n336 = call "StopDaq.vi"("Error in"=w6, "DaqMeasurement"=w8, "DevicesAndSignals"=w7) -> ("Error out"=w16:errorcluster, "DevicesAndSignals"=w15:T1)  [unwired: 7 in]
  n337 = call "DisconnectDevice.vi"("Error in"=w16, "DevicesAndSignals"=w15) -> ("Error out"=w14:errorcluster)  [unwired: 9 in]
  n338 = call <vilib>:"Simple Error Handler.vi"("error in (no error)"=w14) -> ("error out"=w33:errorcluster)  [unwired: 4 in, 4 out]
  n339 = call "DisposeApi.vi"("Error in"=w33) -> ()  [unwired: 10 in, 1 out]
  "VI wird beendet" <- "VI wird ordnungsgemäß beendet, bitte einen Moment Geduld"
  "Numeric" <- 0
